vi "Set Summenformel.vi"(8 "error in (no error)":errorcluster caption="Fehler (Eingang, kein Fehler)", 9 "Summenformel":T2, 10 "Gaskomponente":T1, 11 "SPAN Idx":i32) -> (0 "error out":errorcluster caption="Fehler (Ausgang)")   [LabVIEW 2020, in "Linearisierung v2.lvlib" / "SpanEinstellungen.lvlib"]
uses:
  SpanEinstellungen.lvlib
  Visualisierungs Elemente/String - Eingabefeld.ctl
  Visualisierungs Elemente/Auswahlfeld.ctl
  Aktion FGV SpanEinstellungen.ctl
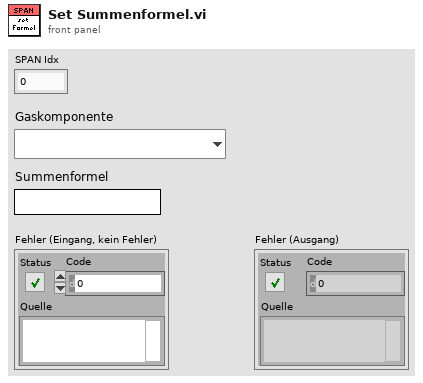
[diagram p1: front panel]
types:
  T1 = typedef "Auswahlfeld.ctl" = u16
  T2 = typedef "String - Eingabefeld.ctl" = string
  T3 = typedef "Linearisierung v2.lvlib/SpanEinstellungen.lvlib/Aktion FGV SpanEinstellungen.ctl" = enum16{"lesen", "schreiben", "laden", "speichern", "RegisterRef", "automatisch", "init", "PDF Params", "Punkte umkehren"}
  T4 = typedef "Linearisierung v2.lvlib/SpanEinstellungen.lvlib/SpanInletCluster.ctl" = cluster{"Span Inlet Active":T5, "Analysator":T6, "Konfig Gasflasche":T5, "Gasflasche":T7, "Gasflaschen Nr.:":string, "Ablaufdatum":timestamp, "Komponenten":T8, "Zeitdauer Stufen":sgl, "Max Fehler":sgl, "Anzahl Stufen":sgl, "Trägergas":T11, "zusätzliche Zeitdauer Erster Punkt":sgl}
  T5 = typedef "System Einstellungen V2.lvlib/Konfig Gasflasche.ctl" = bool
  T6 = typedef "System Einstellungen V2.lvlib/Analysatoren.ctl" = string
  T7 = typedef "System Einstellungen V2.lvlib/Gasflasche Auswahl.ctl" = u16
  T8 = typedef "Linearisierung v2.lvlib/SpanEinstellungen.lvlib/Komponentencluster mit Formel.ctl" = cluster{"Komponente 1":T9, "Komponente 2":T9, "Komponente 3":T9, "Komponente 4":T9, "Komponente 5":T9}
  T9 = typedef "Linearisierung v2.lvlib/SpanEinstellungen.lvlib/Komponentenauswahl mit Formel.ctl" = cluster{"Komponente:":u16, "Summenformel":T2, "Konzentration IST":dbl, "Einheit":T10, "Genauigkeit":dbl}
  T10 = typedef "Linearisierung v2.lvlib/SpanEinstellungen.lvlib/Einheit.ctl" = enum16{"ppm", "%"}
  T11 = typedef "System Einstellungen V2.lvlib/Traegergas.ctl" = string
  T12 = cluster{"Komponenten[0]":T9, "Komponenten[1]":T9, "Komponenten[2]":T9, "Komponenten[3]":T9, "Komponenten[4]":T9}
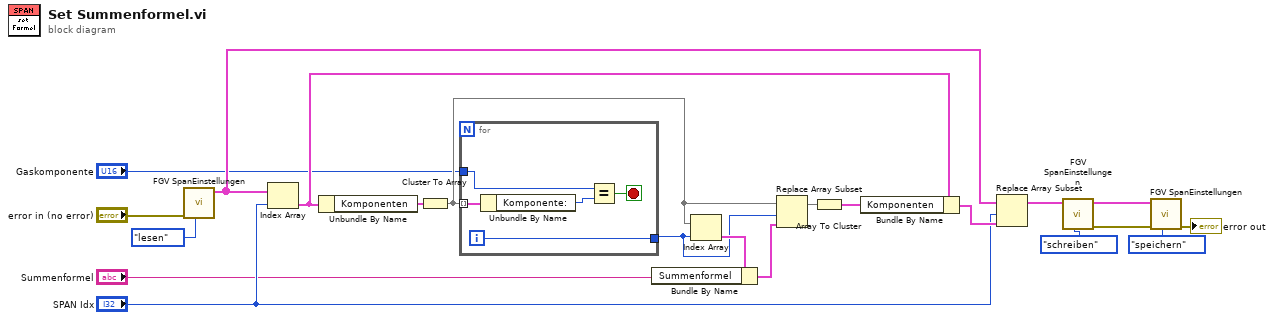
[diagram p0: block diagram]
diagram:
  n1 = call "FGV SpanEinstellungen.vi"("Aktion"=Aktion_FGV_SpanEinstellungen."lesen", "error in (no error)"="error in (no error)") -> ("SpanInletClusterArray out"=w9:T4[])  [unwired: 5 in, 4 out]
  n2 = Index Array(array=w9, index="SPAN Idx") -> (element=w12:T4)
  n3 = Unbundle By Name(w12) -> ("Komponenten"=w17:T8)
  n4 = Cluster To Array(cluster=w17) -> (array=w15:T9[])
  n5 = for {
    tunnel: w15 -> [w26] mode=indexing
    tunnel: "Gaskomponente" -> [w24]
    tunnel: [w22] -> w13
    i -> [w22]
    stop <- w23 stop-if-true
    n6 = Unbundle By Name(w26) -> ("Komponente:"=w25:u16)
    n7 = Equal?(x=w24, y=w25) -> (x = y?=w23:bool)
  }
  n8 = Index Array(array=w15, index=w13) -> (element=w16:T9)
  n9 = Bundle By Name(cluster=w16, "Summenformel"="Summenformel") -> (w14:T9)
  n10 = Replace Array Subset(array=w15, new element=w14, index=w13) -> (w11:T9[])
  n11 = Array To Cluster(array=w11) -> (cluster=w10:T12)
  n12 = Bundle By Name(cluster=w12, "Komponenten"=w10) -> (w8:T4)
  n13 = Replace Array Subset(array=w9, new element=w8, index="SPAN Idx") -> (w7:T4[])
  n14 = call "FGV SpanEinstellungen.vi"("Aktion"=Aktion_FGV_SpanEinstellungen."schreiben", "SpanInletClusterArray in"=w7) -> ("error out"=w19:errorcluster, "SpanInletClusterArray out"=w20:T4[])  [unwired: 5 in, 3 out]
  n15 = call "FGV SpanEinstellungen.vi"("Aktion"=Aktion_FGV_SpanEinstellungen."speichern", "error in (no error)"=w19, "SpanInletClusterArray in"=w20) -> ("error out"=→"error out":errorcluster)  [unwired: 4 in, 4 out]
